vi "Update State Name.vi"(8 "error in (no error)":errorcluster, 9 "New State":string, 10 "State":string, 11 "Channel Ref in":T1 format="%.0x") -> (0 "error out":errorcluster, 3 "Channel Ref out":T1=18446744073709551615 format="%.0x")   [LabVIEW 2017, in "Switch Scripting.lvlib"]
uses:
  Switch Scripting.lvlib
  <vilib>/NI Veristand/Custom Device API/Custom Device Item Ref.ctl
  <vilib>/NI VeriStand/Custom Device API/Custom Device API.lvlib
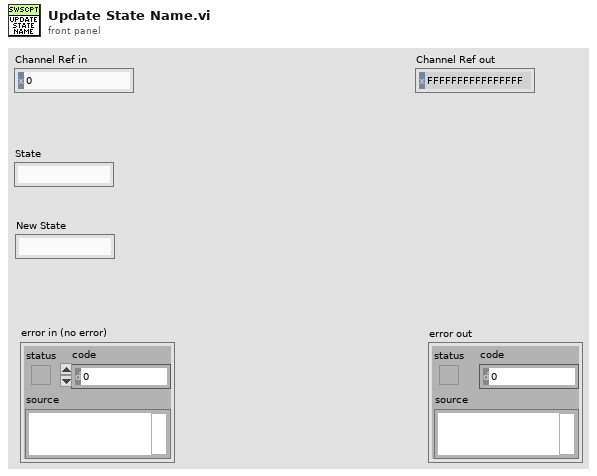
[diagram p1: front panel]
types:
  T1 = typedef "Custom Device API.lvlib/Custom Device Item Ref.ctl" = u64
  T2 = typedef "Switch Scripting.lvlib/Routing State.ctl" = cluster{"name":string, "description":string, "value":i32, "connection list":T3[]}
  T3 = typedef "Switch Scripting.lvlib/Connection.ctl" = cluster{"source":string, "destination":string}
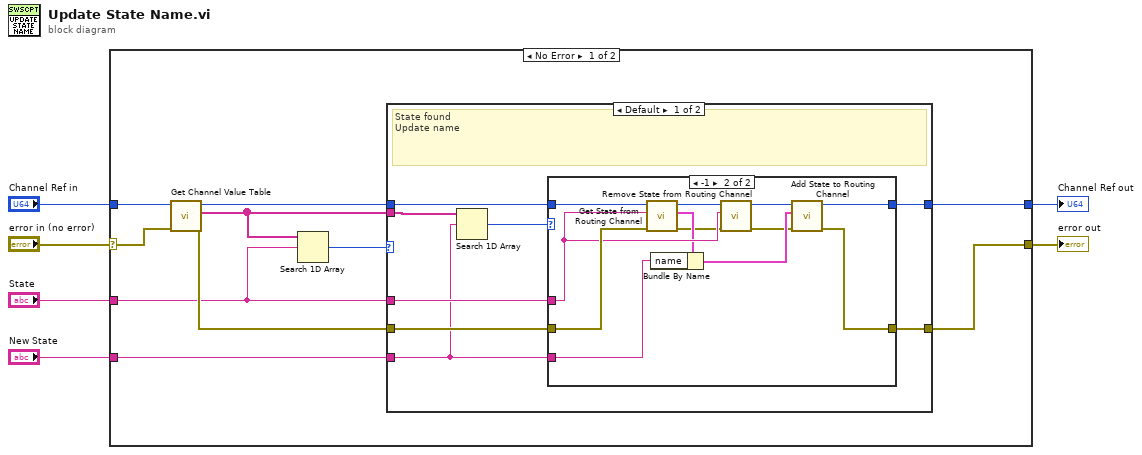
[diagram p0: block diagram]
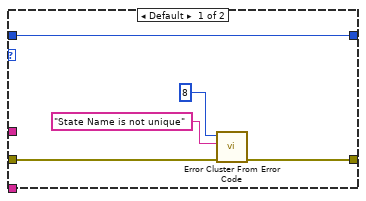
[diagram p2: hidden frame]
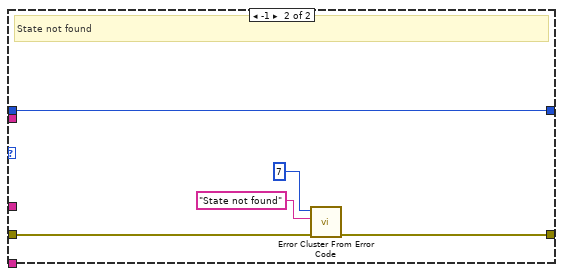
[diagram p3: hidden frame]
diagram:
  n1 = case shown="No Error" "error in (no error)" {
    selector: "error in (no error)" -> [w15 w48]
    tunnel: [w11 w48] -> w2
    tunnel: "Channel Ref in" -> [w16 w47]
    tunnel: [w12 w47] -> w4
    tunnel: "State" -> [w9 _]
    tunnel: "New State" -> [w8 _]
    frame No Error {
      n2 = call "Get Channel Value Table.vi"("error in (no error)"=w15, "Channel Ref in"=w16) -> ("error out"=w13:errorcluster, "States"=w10:string[], "Channel Ref out"=w14:T1)  [unwired: 6 in, 1 out]
      n3 = Search 1D Array(1D array=w10, element=w9) -> (index of element=w7:i32)  [unwired: 1 in]
      n4 = case shown="Default" w7 {
        tunnel: w14 -> [w24 w42]
        tunnel: w13 -> [w23 w44]
        tunnel: [w17 w42] -> w12
        tunnel: [w19 w43] -> w11
        tunnel: w8 -> [w20 _]
        tunnel: w10 -> [w21 _]
        tunnel: w9 -> [w22 _]
        frame Default {
          # "State found\nUpdate name"
          n5 = Search 1D Array(1D array=w21, element=w20) -> (index of element=w18:i32)  [unwired: 1 in]
          n6 = case shown="-1" w18 {
            tunnel: w24 -> [w25 w41]
            tunnel: w23 -> [w27 w40]
            tunnel: w22 -> [_ w39]
            tunnel: w20 -> [_ w37]
            tunnel: [w26 w34] -> w19
            tunnel: [w25 w31] -> w17
            frame Default {
              n7 = call <vilib>:"Error Cluster From Error Code.vi"("error in (no error)"=w27, "error message (\"\")"="State Name is not unique" ("error message (\"\")"), "error code (0)"=8) -> ("error out"=w26:errorcluster)  [unwired: 6 in]
            }
            frame -1 {
              n8 = call "Get State from Routing Channel.vi"("error in (no error)"=w40, "State"=w39, "Channel Ref in"=w41) -> ("error out"=w30:errorcluster, "Routing State"=w38:T2, "Channel Ref out"=w33:T1)  [unwired: 6 in]
              n9 = Bundle By Name(cluster=w38, "name"=w37) -> (w36:T2)
              n10 = call "Remove State from Routing Channel.vi"("error in (no error)"=w30, "State"=w39, "Channel Ref in"=w33) -> ("error out"=w35:errorcluster, "Channel Ref out"=w32:T1)  [unwired: 7 in]
              n11 = call "Add State to Routing Channel.vi"("error in (no error)"=w35, "Routing State"=w36, "Channel Ref in"=w32) -> ("error out"=w34:errorcluster, "Channel Ref out"=w31:T1)  [unwired: 7 in]
            }
          }
        }
        frame -1 {
          # "State not found"
          n12 = call <vilib>:"Error Cluster From Error Code.vi"("error in (no error)"=w44, "error message (\"\")"="State not found" ("error message (\"\")"), "error code (0)"=7) -> ("error out"=w43:errorcluster)  [unwired: 6 in]
        }
      }
    }
    frame Error {
    }
  }
  "Channel Ref out" <- w4
  "error out" <- w2
